vi "Write PWM.vi"(8 "error in (no error)":errorcluster, 10 "PWM":T1 {"PWM Channels"."PWM frequency" items=["1 Hz", "50 Hz", "250 Hz", "500 Hz", "1 kHz", "5 kHz", "10 kHz", "20 kHz"]}, 11 "SD Module in":refnum<class "SD Module.lvclass">) -> (0 "error out":errorcluster, 3 "SD Module out":refnum<class "SD Module.lvclass">)   [LabVIEW 2019, in "Modules.lvlib" / "SD Module.lvclass"]
uses:
  SD Module.lvclass
  Type Defs/PWM.ctl
  Type Defs/PWM Channel.ctl
  SD Module.lvclass/SD Module.ctl
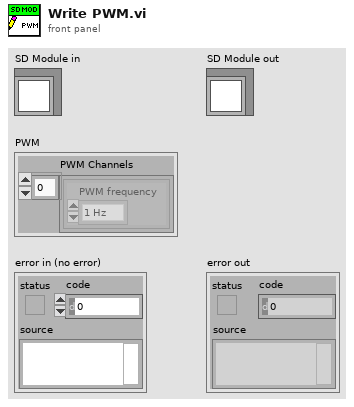
[diagram p1: front panel]
types:
  T1 = typedef "Modules.lvlib/SD Module.lvclass/PWM.ctl" = cluster{"PWM Channels":T2[]}
  T2 = typedef "Modules.lvlib/SD Module.lvclass/PWM Channel.ctl" = cluster{"PWM frequency":u32}
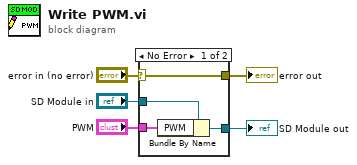
[diagram p0: block diagram]
diagram:
  n1 = case shown="No Error" "error in (no error)" {
    selector: "error in (no error)" -> [w9 w10]
    tunnel: [w9 w10] -> w4
    tunnel: [w7 w11] -> w2
    tunnel: "SD Module in" -> [w8 w11]
    tunnel: "PWM" -> [w6 _]
    frame No Error {
      n2 = Bundle By Name(cluster=w8, "PWM"=w6) -> (w7:refnum<class "SD Module.lvclass">)
    }
    frame Error {
    }
  }
  "error out" <- w4
  "SD Module out" <- w2
